vi "PH_AxisGUI_BaseClass.read Database.vi"(2 "error in (no error)":errorcluster, 3 "DB Entry to read":string) -> (0 "error out":errorcluster, 1 "DB EntriesArray":T1[](array[typedef]))   [LabVIEW 2014, in "PH_AxisGUI_BaseClass.lvlib"]
uses:
  PH_AxisGUI_BaseClass.lvlib
  PH_AxisGUI_BaseClass.Database Entry.ctl
  PH_Stepmotor_BaseClass/PH_Stepmotor_BaseClass.Axis Address.ctl
  PH_Stepmotor_BaseClass/PH_Stepmotor_BaseClass.lvlib
  PH_Common/PH_Common.lvlib
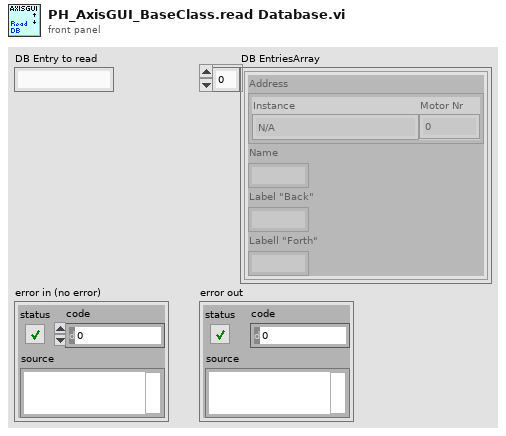
[diagram p1: front panel]
types:
  T1 = typedef "PH_AxisGUI_BaseClass.lvlib/PH_AxisGUI_BaseClass.Database Entry.ctl" = cluster{"Address":T2, "Name":string, "Label \"Back\"":string, "Labell \"Forth\"":string}
  T2 = typedef "PH_Stepmotor_BaseClass.lvlib/PH_Stepmotor_BaseClass.Axis Address.ctl" = cluster{"Instance":string, "Motor Nr":i32}
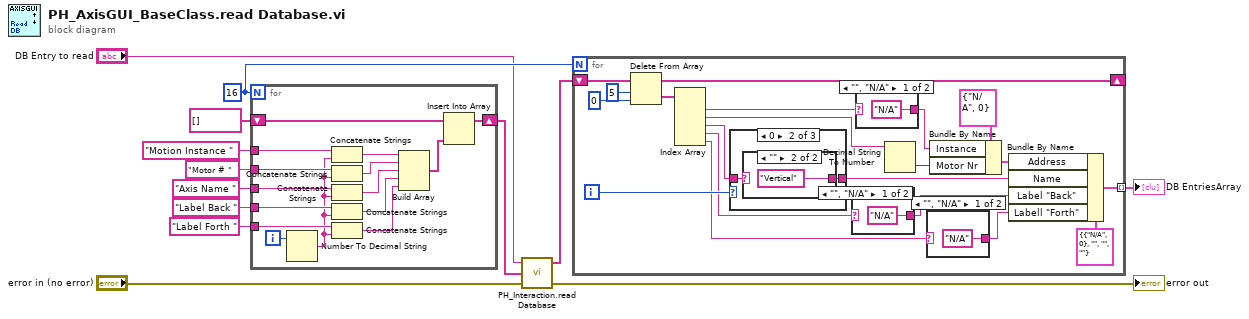
[diagram p0: block diagram]
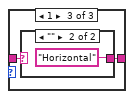
[diagram p6: hidden frame]
diagram:
  w13 = 16
  n1 = for {
    N: w13 -> [_]
    tunnel: "Motion Instance " -> [w27]
    tunnel: "Motor # " -> [w26]
    tunnel: "Axis Name " -> [w25]
    tunnel: "Label Back " -> [w24]
    tunnel: "Label Forth " -> [w23]
    shift-right: [w15] -> w10
    shift-left: string[] [] -> [w14]
    i -> [w28]
    n2 = Number To Decimal String(number=w28) -> (decimal integer string=w22:string)  [unwired: 1 in]
    n3 = Concatenate Strings(w27, w22) -> (w21:string)
    n4 = Concatenate Strings(w26, w22) -> (w20:string)
    n5 = Concatenate Strings(w25, w22) -> (w19:string)
    n6 = Concatenate Strings(w24, w22) -> (w18:string)
    n7 = Concatenate Strings(w23, w22) -> (w17:string)
    n8 = Build Array(w21, w20, w19, w18, w17) -> (w16:string[])
    n9 = Insert Into Array(array=w14, new element=w16) -> (w15:string[])  [unwired: 1 in]
  }
  n10 = call "PH_Interaction.read Database.vi"("error in (no error)"="error in (no error)", "Strings to search for"=w10, "DB Entry to read"="DB Entry to read") -> ("error out"=→"error out":errorcluster, "Values"=w12:string[])  [unwired: 1 in]
  n11 = for {
    N: w13 -> [_]
    tunnel: [w48] -> w11 mode=indexing
    shift-right: [w45] -> _
    shift-left: w12 -> [w46]
    i -> [w35]
    n12 = Delete From Array(array=w46, length=5, index=0) -> (deleted portion=w42:string[], array with subset deleted=w45:string[])
    n13 = Index Array(array=w42) -> (element #1=w37:string, element #2=w39:string, element #3=w34:string, element #4=w31:string, element #5=w32:string)  [unwired: 5 in]
    n14 = case shown="0" w35 {
      tunnel: w34 -> [w53 w55 w59]
      tunnel: [w53 w54 w58] -> w33
      frame Default {
      }
      frame 0 {
        n15 = case shown="\"\"" w55 {
          selector: w55 -> [w56 _]
          tunnel: [w56 "Vertical"] -> w54
          frame Default {
          }
          frame "" {
          }
        }
      }
      frame 1 {
        n16 = case shown="\"\"" w59 {
          selector: w59 -> [w60 _]
          tunnel: [w60 "Horizontal"] -> w58
          frame Default {
          }
          frame "" {
          }
        }
      }
    }
    n17 = case shown="\"\", \"N/A\"" w31 {
      selector: w31 -> [_ w52]
      tunnel: ["N/A" w52] -> w30
      frame "", "N/A" {
      }
      frame Default {
      }
    }
    n18 = case shown="\"\", \"N/A\"" w37 {
      selector: w37 -> [_ w63]
      tunnel: ["N/A" w63] -> w36
      frame "", "N/A" {
      }
      frame Default {
      }
    }
    n19 = Decimal String To Number(string=w39) -> (number=w38:i32)  [unwired: 2 in, 1 out]
    n20 = case shown="\"\", \"N/A\"" w32 {
      selector: w32 -> [_ w50]
      tunnel: ["N/A" w50] -> w29
      frame "", "N/A" {
      }
      frame Default {
      }
    }
    n21 = Bundle By Name(cluster=T2 {"Instance"="N/A", "Motor Nr"=0} ("Address"), "Instance"=w36, "Motor Nr"=w38) -> (w40:T2)
    n22 = Bundle By Name(cluster=T1 {"Address"={"Instance"="N/A", "Motor Nr"=0}, "Name"="", "Label \"Back\""="", "Labell \"Forth\""=""} ("Axis"), "Address"=w40, "Name"=w33, "Label \"Back\""=w30, "Labell \"Forth\""=w29) -> (w48:T1)
  }
  "DB EntriesArray" <- w11
